vi "strings to line.vi"(11 "strings":string[](array[string])) -> (3 "line":T1={"ID"="", "Setpoint"=refnum, "Process Variable"=refnum, "Output"=refnum, "PID gains"={"proportional gain (Kc)"=1.0, "integral time (Ti, min)"=0.01, "derivative time (Td, min)"=0.0}, "output range"={"output high"=100.0, "output low"=-100.0}} {"output range"."output low" format="%.2f"; "output range"."output high" format="%.2f"; "PID gains"."proportional gain (Kc)" format="%.2f"; "PID gains"."integral time (Ti, min)" format="%.2f"})   [LabVIEW 2014, in "Tagbus PID Module editor node.lvclass"]
uses:
  Tagbus PID Module editor node.lvclass
  table line.ctl
  <vilib>/NI/Tag Bus Module Framework/channel/TBM channel.lvclass
  <vilib>/NI/Tag Bus Module Framework/channel/channel classification.ctl
  <vilib>/NI/Tag Bus/tag/Data Type.ctl
  <vilib>/NI/Tag Bus/tag/tag descriptor.lvclass
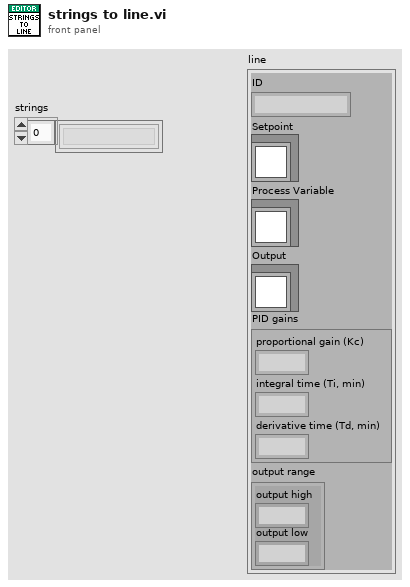
[diagram p1: front panel]
types:
  T1 = typedef "Tagbus PID Module editor node.lvclass/table line.ctl" = cluster{"ID":string, "Setpoint":refnum<class "TBM channel.lvclass">, "Process Variable":refnum<class "TBM channel.lvclass">, "Output":refnum<class "TBM channel.lvclass">, "PID gains":cluster{"proportional gain (Kc)":dbl, "integral time (Ti, min)":dbl, "derivative time (Td, min)":dbl}, "output range":cluster{"output high":dbl, "output low":dbl}}
  T2 = typedef "TBM channel.lvclass/channel classification.ctl" = enum16{"input data", "output data", "processing parameter", "processing result"}
  T3 = typedef "tag bus.lvlib/tag descriptor.lvclass/Data Type.ctl" = enum16{"Double", "Single", "I64", "I32", "I16", "I8", "U64", "U32", "U16", "U8", "Boolean", "String", "Array of Double", "Array of Single", "Array of I64", "Array of I32", "Array of I16", "Array of I8", "Array of U64", "Array of U32", "Array of U16", "Array of U8", "Array of Boolean", "Array of String"}
  T4 = cluster{"proportional gain (Kc)":dbl, "integral time (Ti, min)":dbl, "derivative time (Td, min)":dbl}
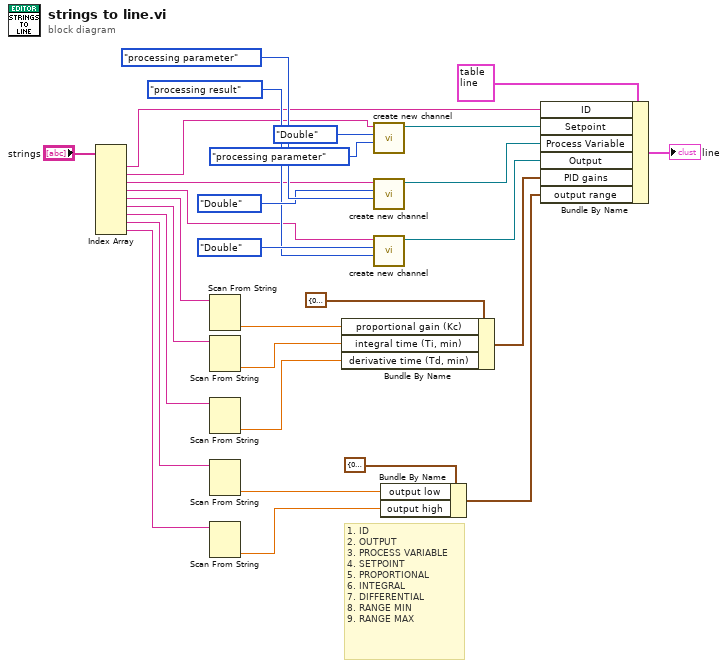
[diagram p0: block diagram]
diagram:
  # "1. ID\n2. OUTPUT\n3. PROCESS VARIABLE\n4. SETPOINT\n5. PROPORTIONAL\n6. INTEGRAL\n7. DIFFERENTIAL\n8. RANGE MIN\n9. RANGE MAX"
  n1 = Index Array(array="strings") -> (element #1=w7:string, element #2=w6:string, element #3=w5:string, element #4=w4:string, element #5=w8:string, element #6=w27:string, element #7=w26:string, element #8=w17:string, element #9=w16:string)  [unwired: 9 in]
  n2 = Scan From String(input string=w8) -> (output 1=w24:dbl)  [unwired: 4 in, 3 out]
  n3 = Scan From String(input string=w27) -> (output 1=w23:dbl)  [unwired: 4 in, 3 out]
  n4 = Scan From String(input string=w26) -> (output 1=w22:dbl)  [unwired: 4 in, 3 out]
  n5 = Scan From String(input string=w17) -> (output 1=w19:dbl)  [unwired: 4 in, 3 out]
  n6 = Scan From String(input string=w16) -> (output 1=w18:dbl)  [unwired: 4 in, 3 out]
  n7 = Bundle By Name(cluster=T4 {"proportional gain (Kc)"=0.0, "integral time (Ti, min)"=0.0, "derivative time (Td, min)"=0.0} ("PID gains"), "proportional gain (Kc)"=w24, "integral time (Ti, min)"=w23, "derivative time (Td, min)"=w22) -> (w21:T4)
  n8 = call <vilib>:"create new channel.vi"("channel classification"=channel_classification."processing parameter", "data type"=Data_Type."Double", "channel name"=w6) -> ("channel"=w3:refnum<class "TBM channel.lvclass">)  [unwired: 8 in]
  n9 = call <vilib>:"create new channel.vi"("channel classification"=channel_classification."processing parameter", "data type"=Data_Type."Double", "channel name"=w5) -> ("channel"=w2:refnum<class "TBM channel.lvclass">)  [unwired: 8 in]
  n10 = call <vilib>:"create new channel.vi"("channel classification"=channel_classification."processing result", "data type"=Data_Type."Double", "channel name"=w4) -> ("channel"=w1:refnum<class "TBM channel.lvclass">)  [unwired: 8 in]
  n11 = Bundle By Name(cluster=cluster{"output high":dbl, "output low":dbl} {"output high"=0.0, "output low"=0.0} ("output range"), "output low"=w19, "output high"=w18) -> (w15:cluster{"output high":dbl, "output low":dbl})
  n12 = Bundle By Name(cluster=T1 {"ID"="", "Setpoint"=refnum, "Process Variable"=refnum, "Output"=refnum, "PID gains"={"proportional gain (Kc)"=1.0, "integral time (Ti, min)"=0.01, "derivative time (Td, min)"=0.0}, "output range"={"output high"=100.0, "output low"=-100.0}} ("line"), "ID"=w7, "Setpoint"=w3, "Process Variable"=w2, "Output"=w1, "PID gains"=w21, "output range"=w15) -> (→"line":T1)
